vi "labview_analog_voltage_single_io.vi"() -> ()   [LabVIEW 2021]
uses:
  <vilib>/DAQmx/write.llb/DAQmx Write (Analog DBL 1Chan 1Samp).vi
  <vilib>/DAQmx/read.llb/DAQmx Read (Analog DBL 1Chan 1Samp).vi
  <vilib>/DAQmx/miscellaneous.llb/DAQmx Fill In Error Info.vi
panel:
  in  "stop":bool
  out "AI [V]":dbl(knob) scale=0.0..5.0
  in  "AO [V]":dbl(slide) scale=0.0..5.0
  # "Analog voltage single I/O channels with NI USB-6008"
  # "Finn Aakre Haugen (finn.haugen@usn.no)"
  # "02.12 2017"
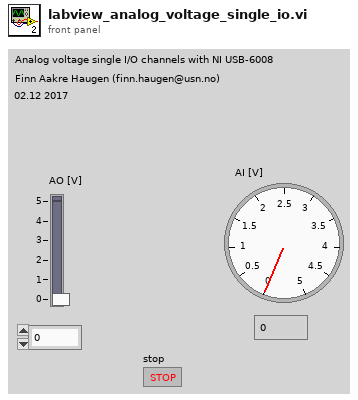
[diagram p1: front panel]
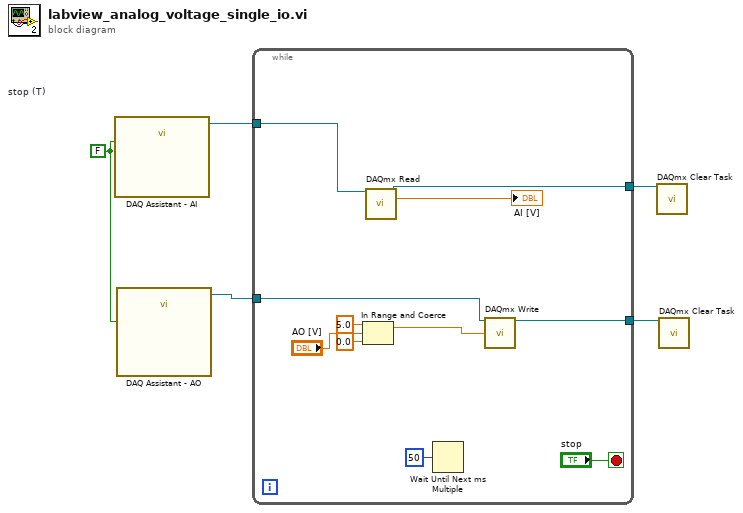
[diagram p0: block diagram]
diagram:
  w5 = FALSE  # stop (T)
  n1 = call "DAQ Assistant - AI"("stop (T)"=w5) -> ("task out"=w3:refnum<k21>)  [unwired: 3 in, 15 out]
  n2 = call "DAQ Assistant - AO"("stop (T)"=w5) -> ("task out"=w4:refnum<k21>)  [unwired: 4 in, 14 out]
  n3 = while {
    tunnel: w3 -> [w15]
    tunnel: w4 -> [w11]
    tunnel: [w7] -> w2
    tunnel: [w6] -> w1
    stop <- "stop" stop-if-true
    n4 = In Range and Coerce(upper limit=5.0, x="AO [V]", lower limit=0.0) -> (coerced(x)=w10:dbl)  [unwired: 1 out]
    n5 = call-poly <vilib>:"DAQmx Read.vi"("task/channels in"=w15) -> ("task out"=w7:refnum<k21>, "data"=→"AI [V]":dbl)  [unwired: 1 in, 12 out]
    n6 = Wait Until Next ms Multiple(millisecond multiple=u32 50) -> ()  [unwired: 1 out]
    n7 = call-poly <vilib>:"DAQmx Write.vi"("task/channels in"=w11, "data"=w10) -> ("task out"=w6:refnum<k21>)  [unwired: 2 in, 11 out]
  }
  n8 = call <vilib>:"DAQmx Clear Task.vi"("task in"=w2) -> ()  [unwired: 14 in, 1 out]
  n9 = call <vilib>:"DAQmx Clear Task.vi"("task in"=w1) -> ()  [unwired: 14 in, 1 out]
